vi "startClosedLoopScan.vi"(8 "error in (no error)":errorcluster, 9 "Scan Settings":T1={"Amplitude Scan Settings"={"Start Value"=1.0, "Stop Value"=1.0, "Steps"=2}, "Rate Scan Settings"=[], "Sample Count"=0, "Iterations"=60.0, "Amplitude"=0.0, "Offset"=0.0, "Frequency"=0.0, "Waveform"=enum."Sine", "F1"=0.0, "F2"=0.0, "Duty Cycle"=0.0, "ILC Rate"=0.0, "Operator"="", "Scan Name"="", "Notes"="", "Ramp Time"=0.0, "Hold Time"=0.0, "Settling Time"=0.0, "Control Mode"=enum."PSV", "FCV Rate"=0.0} {"Amplitude Scan Settings"."Stop Value" format="%.3f"; "Amplitude Scan Settings"."Start Value" format="%.3f"}, 10 "Model in":refnum<class "Model.lvclass">, 11 "WaitForUserInputState in":refnum<class "WaitForUserInputState.lvclass">) -> (0 "error out":errorcluster, 2 "Model out":refnum<class "Model.lvclass">, 3 "WaitForUserInputState out":refnum<class "WaitForUserInputState.lvclass">)   [LabVIEW 2015, in "WaitForUserInputState.lvclass"]
uses:
  WaitForUserInputState.lvclass
  Model/Model/Model.lvclass
  Typedefs/Scan Settings.ctl
  Typedefs/Test Values.ctl
  <userlib>/Common/ILC/Configuration/Scan Rates.ctl
  Typedefs/Waveform.ctl
  Typedefs/ControlMode.ctl
  Typedefs/StateSelector.ctl
  Model/Model/Model.lvclass/Model.ctl
  Typedefs/FAMTTypedefs.lvlib
  <userlib>/Common/ILC/Configuration/ILCConfiguration.lvlib
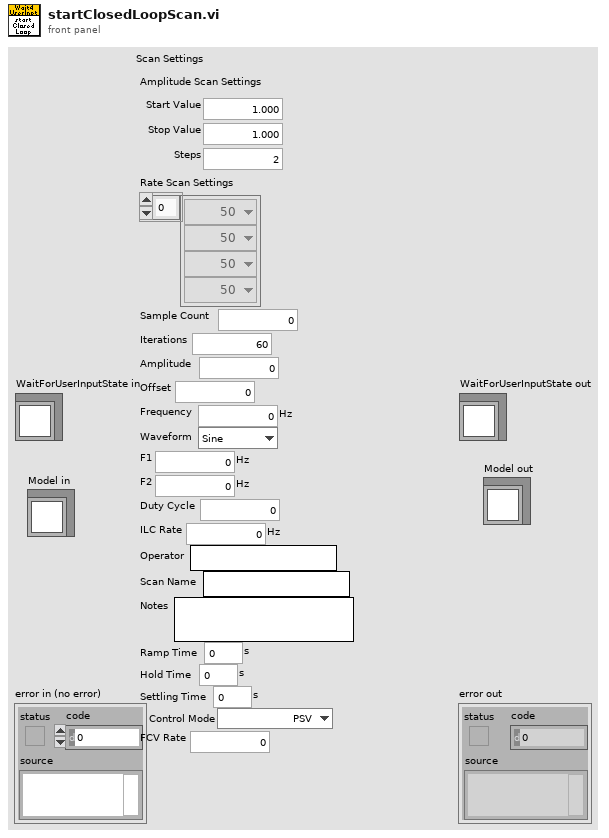
[diagram p1: front panel]
types:
  T1 = typedef "FAMTTypedefs.lvlib/Scan Settings.ctl" = cluster{"Amplitude Scan Settings":T2, "Rate Scan Settings":T3[], "Sample Count":u32, "Iterations":dbl, "Amplitude":dbl, "Offset":dbl, "Frequency":dbl[unit], "Waveform":T4, "F1":dbl[unit], "F2":dbl[unit], "Duty Cycle":dbl, "ILC Rate":dbl[unit], "Operator":string, "Scan Name":string, "Notes":string, "Ramp Time":dbl[unit], "Hold Time":dbl[unit], "Settling Time":dbl[unit], "Control Mode":T5, "FCV Rate":dbl}
  T2 = typedef "FAMTTypedefs.lvlib/Test Values.ctl" = cluster{"Start Value":dbl, "Stop Value":dbl, "Steps":u16}
  T3 = typedef "ILCCommon.lvlib/ILCConfiguration.lvlib/Scan Rates.ctl" = enum16{"50", "60", "100", "120", "200", "240", "300", "400", "480", "600", "1200", "2400", "4800"}
  T4 = typedef "FAMTTypedefs.lvlib/Waveform.ctl" = enum16{"Sine", "Triangle", "Square", "Sawtooth", "Chirp", "Gaussian", "Trapezoid"}
  T5 = typedef "FAMTTypedefs.lvlib/ControlMode.ctl" = enum16{"PSV", "FCV", "Both"}
  T6 = typedef "FAMTTypedefs.lvlib/StateSelector.ctl" = enum16{"OfflineState", "FaultState", "StandbyState", "DisabledState", "EnabledState", "WaitForUserInputState", "PerformOpenLoopScanState", "PerformClosedLoopScanState"}
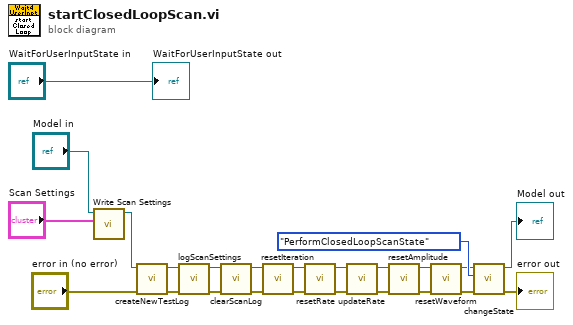
[diagram p0: block diagram]
diagram:
  n1 = call "Write Scan Settings.vi"("Scan Settings"="Scan Settings", "Model in"="Model in") -> ("Model out"=w16:refnum<class "Model.lvclass">)  [unwired: 9 in]
  n2 = call "createNewTestLog.vi"("error in (no error)"="error in (no error)", "Model in"=w16) -> ("error out"=w12:errorcluster, "Model out"=w15:refnum<class "Model.lvclass">)  [unwired: 8 in]
  n3 = call "logScanSettings.vi"("error in (no error)"=w12, "Model in"=w15) -> ("error out"=w11:errorcluster, "Model out"=w14:refnum<class "Model.lvclass">)  [unwired: 8 in]
  n4 = call "clearScanLog.vi"("error in (no error)"=w11, "Model in"=w14) -> ("error out"=w2:errorcluster, "Model out"=w1:refnum<class "Model.lvclass">)  [unwired: 8 in]
  n5 = call "resetIteration.vi"("error in (no error)"=w2, "Model in"=w1) -> ("error out"=w10:errorcluster, "Model out"=w19:refnum<class "Model.lvclass">)  [unwired: 8 in]
  n6 = call "resetRate.vi"("error in (no error)"=w10, "Model in"=w19) -> ("error out"=w9:errorcluster, "Model out"=w18:refnum<class "Model.lvclass">)  [unwired: 8 in]
  n7 = call "updateRate.vi"("error in (no error)"=w9, "Model in"=w18) -> ("error out"=w8:errorcluster, "Model out"=w17:refnum<class "Model.lvclass">)  [unwired: 8 in]
  n8 = call "resetAmplitude.vi"("error in (no error)"=w8, "Model in"=w17) -> ("error out"=w6:errorcluster, "Model out"=w3:refnum<class "Model.lvclass">)  [unwired: 8 in]
  n9 = call "resetWaveform.vi"("error in (no error)"=w6, "Model in"=w3) -> ("error out"=w5:errorcluster, "Model out"=w4:refnum<class "Model.lvclass">)  [unwired: 8 in]
  n10 = call "changeState.vi"("error in (no error)"=w5, "State:"=StateSelector."PerformClosedLoopScanState", "Model in"=w4) -> ("error out"=→"error out":errorcluster, "Model out"=→"Model out":refnum<class "Model.lvclass">)  [unwired: 7 in]
  "WaitForUserInputState out" <- "WaitForUserInputState in"
